vi "Voltmeter.vi"() -> ()   [LabVIEW 2017]
uses:
  <vilib>/Instr/_visa.llb/VISA Configure Serial Port (Instr).vi
panel:
  out "V":dbl
  in  "?":bool
  out "Warning: \nVoltge > 4.5 V":bool
  out "Voltmeter":dbl(knob) scale=0.0..10.0
  in  "VISA resource name":refnum<visa-resource-name>
  in  "Channel":i32
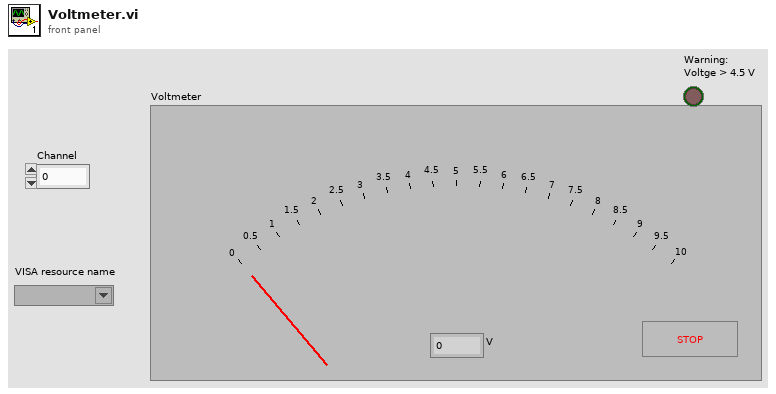
[diagram p1: front panel]
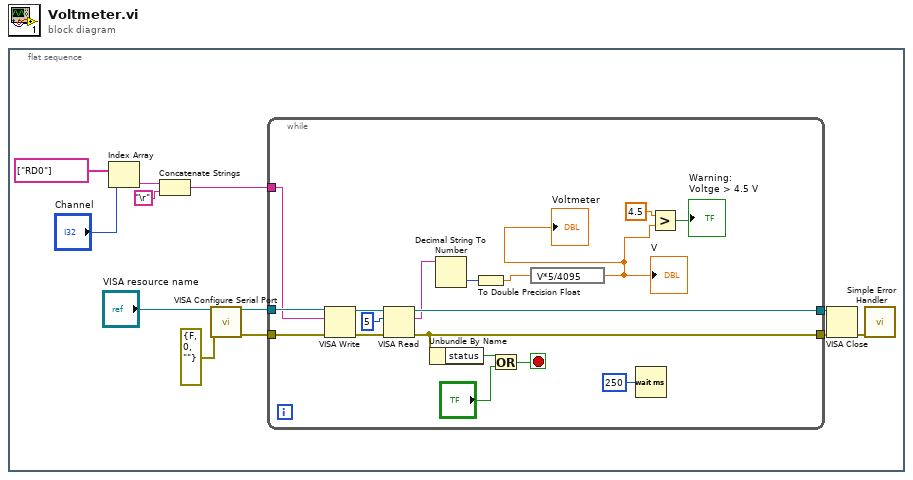
[diagram p0: block diagram]
diagram:
  n1 = flat-sequence {
    frame #0 {
      n2 = Index Array(array=string[] ["RD0"], index="Channel") -> (element=w10:string)
      n3 = Concatenate Strings(w10, "\r") -> (w8:string)
      n4 = call-poly "VISA Configure Serial Port"("VISA resource name"="VISA resource name", "error in (no error)"=errorcluster {"status"=FALSE, "code"=0, "source"=""}) -> ("VISA resource name out"=w4:refnum<visa-resource-name>, "error out"=w5:errorcluster)  [unwired: 12 in]
      n5 = while {
        tunnel: w8 -> [w28]
        tunnel: w5 -> [w30]
        tunnel: w4 -> [w29]
        tunnel: [w22] -> w3
        tunnel: [w24] -> w2
        stop <- w20 stop-if-true
        n6 = VISA Write(VISA resource name=w29, write buffer=w28, error in (no error)=w30) -> (VISA resource name out=w26:refnum<visa-resource-name>, error out=w27:errorcluster)  [unwired: 1 out]
        n7 = VISA Read(VISA resource name=w26, byte count=5, error in (no error)=w27) -> (VISA resource name out=w24:refnum<visa-resource-name>, read buffer=w19:string, error out=w22:errorcluster)  [unwired: 1 out]
        n8 = Unbundle By Name(w22) -> ("status"=w21:bool)
        n9 = Decimal String To Number(string=w19) -> (number=w18:i32)  [unwired: 2 in, 1 out]
        n10 = To Double Precision Float(number=w18) -> (double precision float=w17:dbl)
        n11 = Or(x=w21, y="?") -> (x .or. y?=w20:bool)
        n12 = expression code="V*5/4095"(w17) -> (w15:dbl)
        "V" <- w15
        "Voltmeter" <- w15
        n13 = Wait (ms)(milliseconds to wait=u32 250) -> ()  [unwired: 1 out]
        n14 = Greater?(x=4.5, y=w15) -> (0:→"Warning: \nVoltge > 4.5 V":bool)
      }
      n15 = VISA Close(VISA resource name=w2, error in (no error)=w3) -> (error out=w1:errorcluster)
      n16 = call <vilib>:"Simple Error Handler.vi"("error in (no error)"=w1) -> ()  [unwired: 4 in, 5 out]
    }
  }
